vi "GetRecord.vi"(8 "error in (no error)":errorcluster, 9 "Label":string, 10 "Task":string, 11 "DAQ_Module in":refnum<class "DAQ_Module.lvclass">) -> (0 "error out":errorcluster, 2 "RecordData":T1 {"StopTime" format="%<%x %.3X>T"; "StartTime" format="%<%x %.3X>T"}, 3 "DAQ_Module out":refnum<class "DAQ_Module.lvclass">)   [LabVIEW 2025, in "DAQ_Module.lvlib" / "DAQ_Module.lvclass"]
uses:
  DAQ_Module.lvclass
  DAQ_Abstr/Task_Abstr/Task_Abstr/WaveformData.ctl
  DAQ_Module.lvclass/DAQ_Module.ctl
  DAQ_Abstr/Task_Abstr/Task_Abstr/Task_Abstr.lvclass
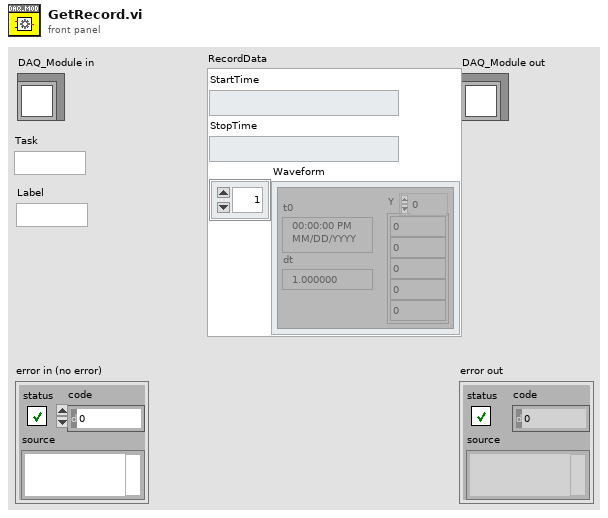
[diagram p1: front panel]
types:
  T1 = typedef "Task_Abstr.lvlib/Task_Abstr.lvclass/WaveformData.ctl" = cluster{"StartTime":timestamp, "StopTime":timestamp, "Waveform":waveform(dbl)[]}
  T2 = typedef "Task_Abstr.lvlib/Task_Abstr.lvclass/DataContainer.ctl" = map{string, T1}
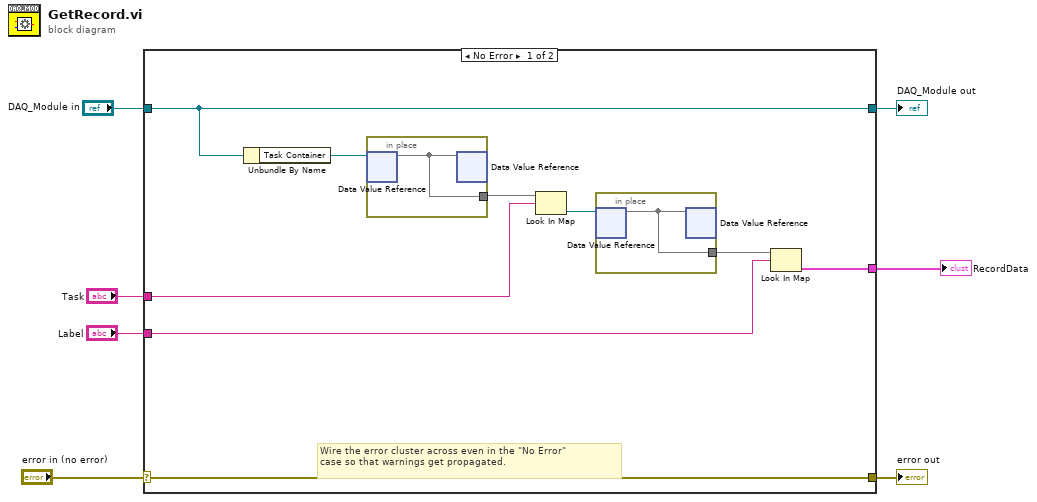
[diagram p0: block diagram]
diagram:
  n1 = case shown="No Error" "error in (no error)" {
    selector: "error in (no error)" -> [w16 w20]
    tunnel: [w16 w20] -> w6
    tunnel: [w15 w19] -> w4
    tunnel: "DAQ_Module in" -> [w15 w19]
    tunnel: "Task" -> [w12 _]
    tunnel: "Label" -> [w9 _]
    tunnel: [w8 _] -> w1
    frame No Error {
      # "Wire the error cluster across even in the \"No Error\"\ncase so that warnings get propagated."
      n2 = Unbundle By Name(w15) -> ("Task Container"=w14:refnum<data-value>)
      n3 = in-place {
        in-place-border: [w18] -> w13
        n4 = in-place-dvr #1(w14) -> (w18:map{string, refnum<data-value>})  [unwired: 1 out]
        n5 = in-place-dvr #1(w18) -> ()  [unwired: 2 out]
      }
      n6 = Look In Map(map=w13, key=w12) -> (value=w11:refnum<data-value>)  [unwired: 1 in, 1 out]
      n7 = in-place {
        in-place-border: [w17] -> w10
        n8 = in-place-dvr #2(w11) -> (w17:T2)  [unwired: 1 out]
        n9 = in-place-dvr #2(w17) -> ()  [unwired: 2 out]
      }
      n10 = Look In Map(map=w10, key=w9) -> (value=w8:T1)  [unwired: 1 in, 1 out]
    }
    frame Error {
    }
  }
  "error out" <- w6
  "DAQ_Module out" <- w4
  "RecordData" <- w1
